vi "REPORT_OPRTN_filter_records.vi"(9 "REPORT_DATES_filters":T1={"order_selection"=enum."new_to_old", "last_status"=""}, 10 "operations_statuses":T2[](array[typedef]), 11 "operations":string[][](array[string])) -> (2 "record_statuses":T2[](array[typedef]), 3 "ItemNames":string[][](array[string]))   [LabVIEW 2019]
uses:
  DATES/typedef/REPORT_DATES_statuses.ctl
  typedef/REPORT_OPRTN_filters.ctl
  <userlib>/_OpenG.lib/array/array.llb/Reverse 2D Array (String)__ogtk.vi
  <userlib>/_OpenG.lib/array/array.llb/Filter 1D Array with Scalar (String)__ogtk.vi
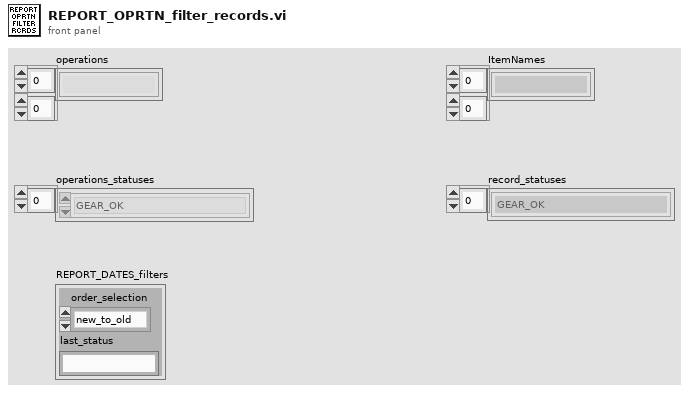
[diagram p1: front panel]
types:
  T1 = typedef "REPORT_OPRTN_filters.ctl" = cluster{"order_selection":enum32{"old_to_new", "new_to_old"}, "last_status":string}
  T2 = typedef "REPORT_DATES_statuses.ctl" = enum16{"GEAR_OK", "GEAR_NOK", "GEAR_interrupted", "GEAR_in_operation", "GEAR_unexpected"}
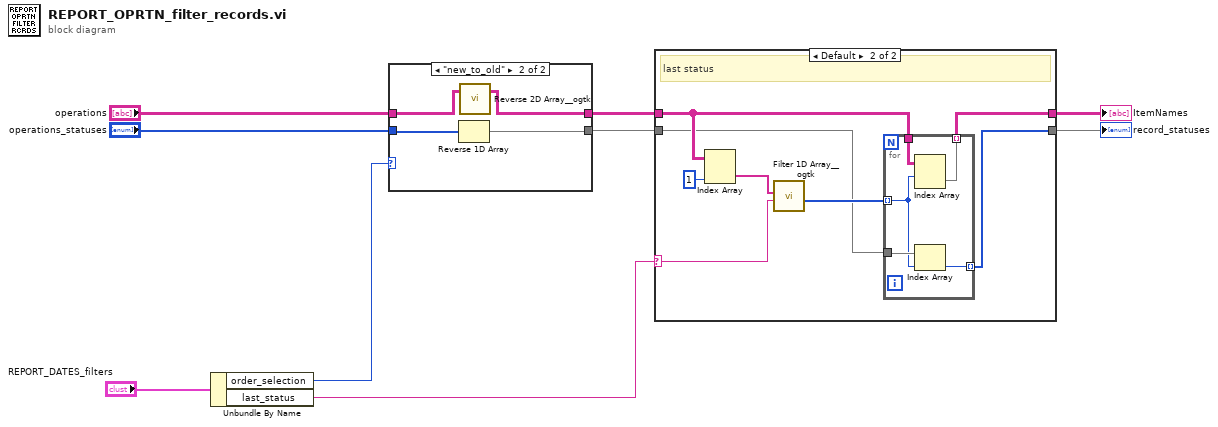
[diagram p0: block diagram]
diagram:
  n1 = Unbundle By Name("REPORT_DATES_filters") -> ("order_selection"=w6:enum32{"old_to_new", "new_to_old"}, "last_status"=w3:string)
  n2 = case shown="\"new_to_old\"" w6 {
    tunnel: "operations" -> [w11 w13]
    tunnel: [w11 w12] -> w2
    tunnel: "operations_statuses" -> [w10 w15]
    tunnel: [w10 w14] -> w1
    frame "old_to_new" {
    }
    frame "new_to_old" {
      n3 = Reverse 1D Array(array=w15) -> (reversed array=w14:T2[])
      n4 = call-poly <userlib>:"Reverse 2D Array__ogtk.vi"("Array"=w13) -> ("Reversed Array"=w12:string[][])  [unwired: 2 in]
    }
  }
  n5 = case shown="Default" w3 {
    selector: w3 -> [_ w25]
    tunnel: [w17 w22] -> w5
    tunnel: w2 -> [w17 w20]
    tunnel: w1 -> [w16 w19]
    tunnel: [w16 w18] -> w4
    frame "ALL" {
      # "last status"
    }
    frame Default {
      # "last status"
      n6 = Index Array(array=w20, index (col)=1 ("disabled index (col)")) -> (element=w23:string[])  [unwired: 1 in]
      n7 = call-poly <userlib>:"Filter 1D Array__ogtk.vi"("items to filter"=w25, "array"=w23) -> ("filtered item indices"=w21:i32[])  [unwired: 4 in, 1 out]
      n8 = for {
        tunnel: w20 -> [w30]
        tunnel: w21 -> [w27] mode=indexing
        tunnel: [w29] -> w22 mode=indexing
        tunnel: w19 -> [w28]
        tunnel: [w26] -> w18 mode=indexing
        n9 = Index Array(array=w30, index (row)=w27) -> (element=w29:string[])  [unwired: 1 in]
        n10 = Index Array(array=w28, index=w27) -> (element=w26:T2)
      }
    }
  }
  "ItemNames" <- w5
  "record_statuses" <- w4
